vi "hello-vi.vi"() -> ()   [LabVIEW 2020]
uses:
  controls/APC_ControlSettings.ctl
  controls/APC_PIDcontrolSettings.ctl
panel:
  out "System State 2":i8
  in  "stop":bool
  out "Client Connected":bool=TRUE
  out "Telemetry seq":i32
  out "Lines received":i32
  out "Last received":string
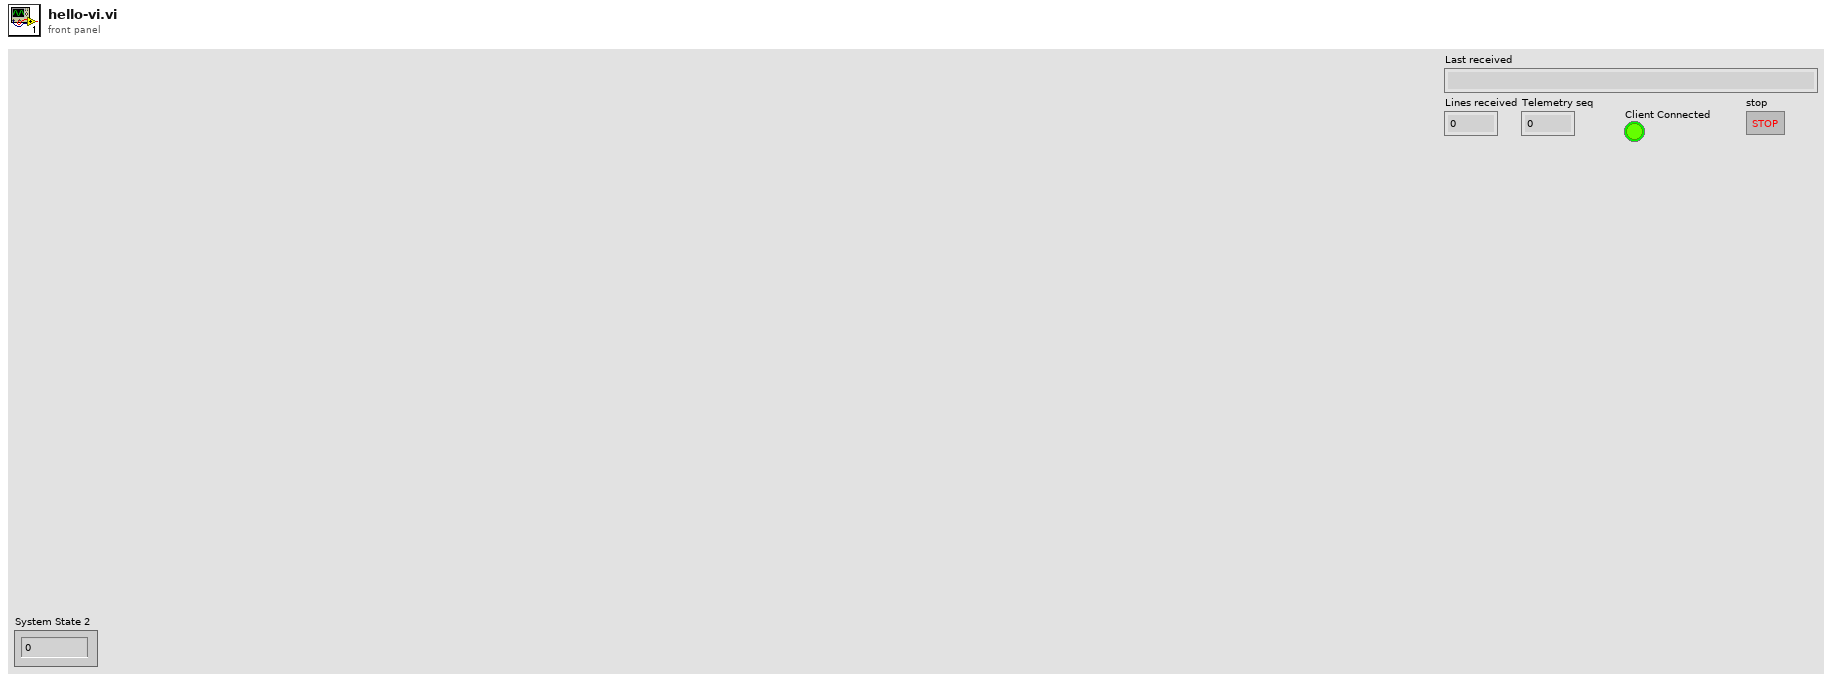
[diagram p1: front panel]
types:
  T1 = enum16{"Standard", "Buffered", "CRLF", "Immediate"}
  T2 = typedef "APC_ControlSettings.ctl" = cluster{"Spark advance [CADBTDC]":dbl, "Pref":dbl, "O2ref":dbl, "DI advance [CADBTDC]":dbl, "DI duration [ms] ":dbl, "CO2ref":dbl, "PFI duration [ms]":dbl, "IMEP ref":dbl, "Speed ref":dbl, "IGN enable":bool, "DI enable":bool, "CL PFI\n lambda":bool, "CL PFI\nIMEP":bool, "Activate\ncylinder":bool[], "Force idling":bool, "Force motoring":bool, "ETP resync":bool, "Requested mode":i8, "Clear Sync Errors":bool, "toggle TDC":bool, "l ref":dbl, "PID control references":T3, "CA50setpoint [CADATDC]":dbl, "CA50 control":bool, "Knock control":bool, "CLEAR EMERGENCY STOP":bool, "EMERGENCY STOP":bool}
  T3 = typedef "APC_PIDcontrolSettings.ctl" = cluster{"NG":bool, "Ar":bool, "O2":bool, "Intake vent":bool, "Cross vent":bool, "Exhaust vent":bool, "NG control mode":u8, "NG-FC-001-REF":dbl, "WF-OA-002-REF":dbl, "IMEP-REF":dbl, "Nm-REF":dbl, "Ar control mode":u8, "AR-PC-002-REF":dbl, "WF-PT-004-REF":dbl, "O2 control mode":u8, "O2-FC-001-REF":dbl, "WF-OA-001-REF":dbl, "Tcoolant control  mode":u8, "EC-FC-001-REF":dbl, "EC-TT-001-REF":dbl, "Texh control mode":u8, "SW-FC-004-REF":dbl, "SW-FT-002-REF":dbl, "WF-TT-004-REF":dbl, "Toil control mode":u8, "SW-FC-009-REF":dbl, "SW-FT-004-REF":dbl, "EO-TT-001-REF":dbl, "AIC201_CO2_ConcTarget":dbl, "O2_FF_NG":bool, "Dyno control mode":u8, "Membrane control mode":u8, "AR-FT-001-REF":dbl, "MTR modbus floats":sgl[], "MTR modbus u16":u16[], "MTR HB":bool, "PC_HB":bool, "EMERGENCY STOP":bool}
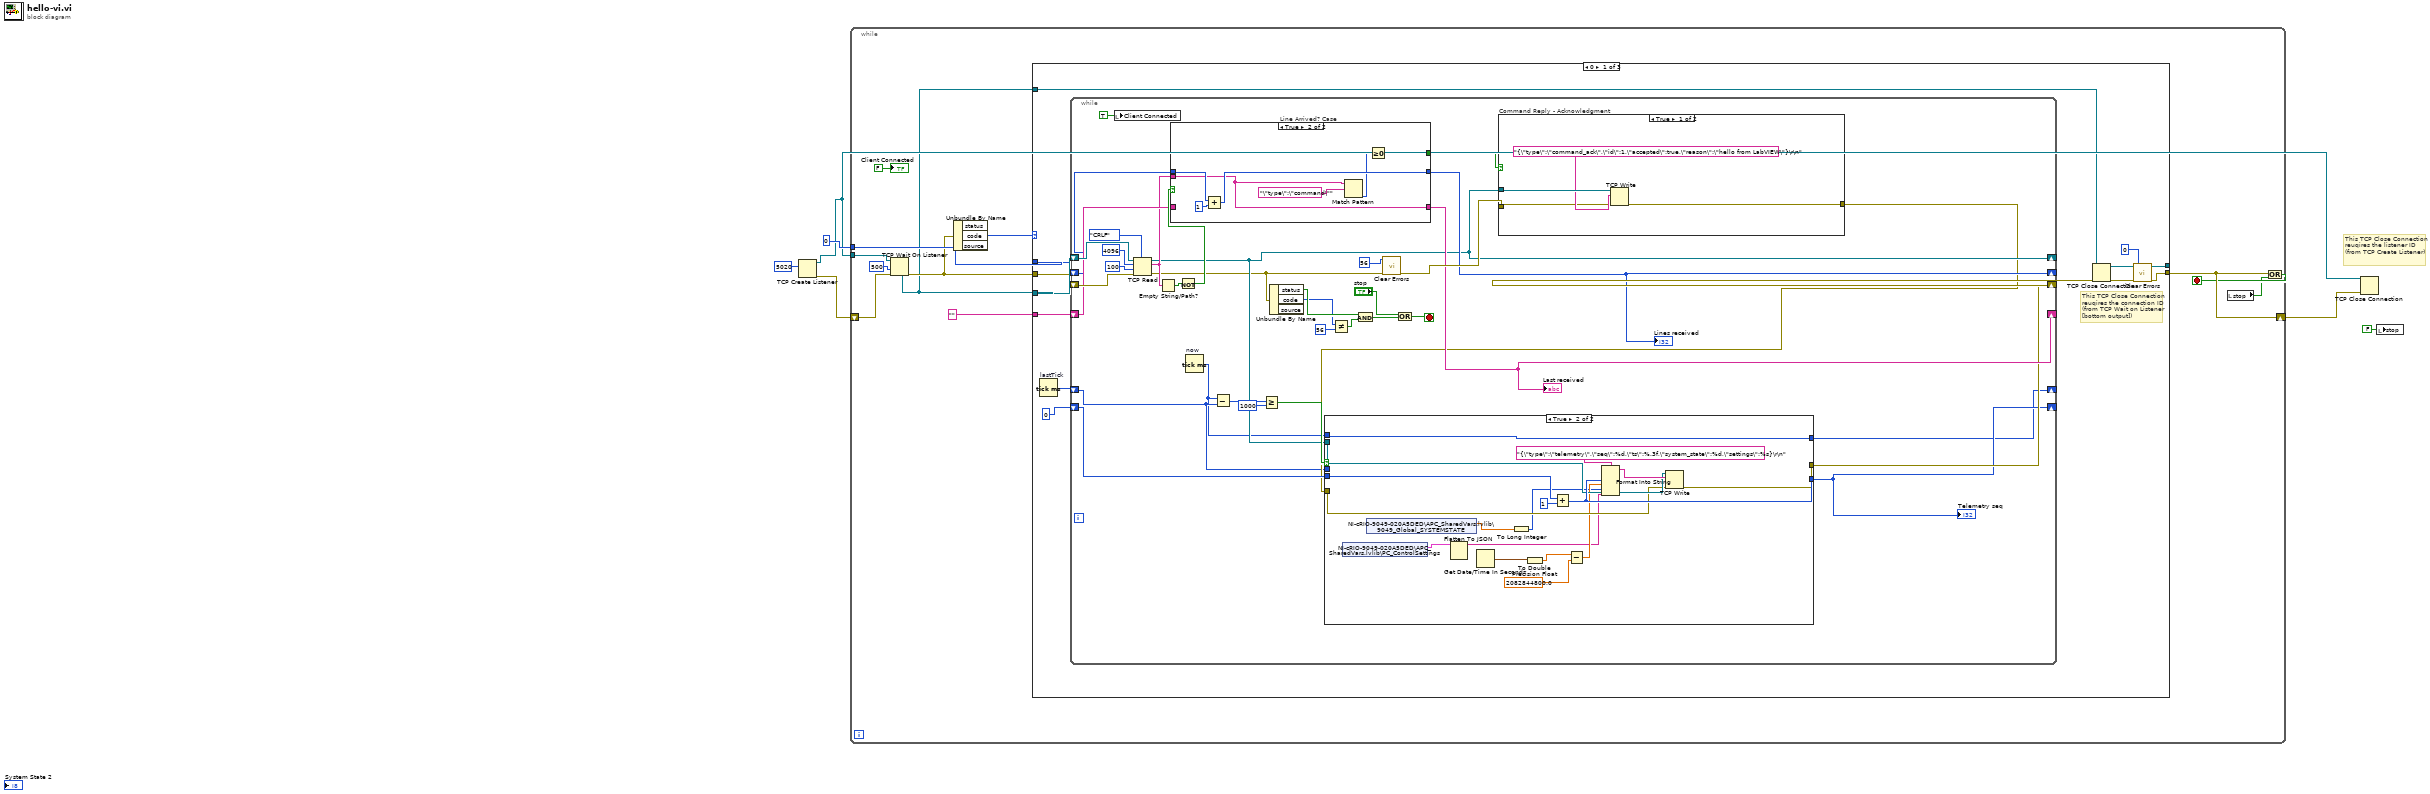
[diagram p0: block diagram]
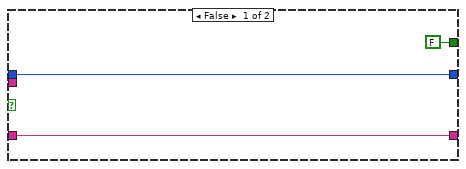
[diagram p3: hidden frame]
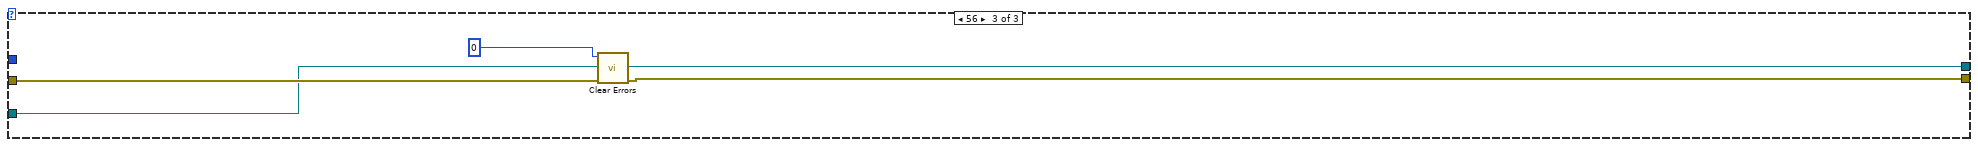
[diagram p6: hidden frame]
diagram:
  # "This TCP Close Connection reuqires the listener ID (from TCP Create Listener)"
  n1 = TCP Create Listener(10:u16 5020 ("port")) -> (0:w4:errorcluster, 3:w1:refnum<k5>)  [unwired: 4 in, 1 out]
  n2 = while {
    tunnel: 0 ("Lines received") -> [w17]
    shift-right: [w12] -> w3
    shift-left: w4 -> [w16]
    tunnel: w1 -> [w9]
    stop <- w11 stop-if-true
    n3 = TCP Wait On Listener(8:w16, 9:500 ("timeout ms (wait forever: -1)"), 11:w9) -> (0:w14:errorcluster, 4:w8:refnum<k5>)  [unwired: 1 in, 3 out]
    n4 = Unbundle By Name(w14) -> ("code"=w13:i32)  [unwired: 2 out]
    n5 = case shown="0" w13 {
      tunnel: w8 -> [w30 w102 w103]
      tunnel: w17 -> [w29 _ _]
      tunnel: [w23 w102 w103] -> _
      tunnel: [w24 w101 w104] -> w12
      tunnel: w14 -> [w28 w101 w105]
      tunnel: w8 -> [w22 _ _]
      tunnel: "" -> [w21 _ _]
      frame 0 {
        # "This TCP Close Connection reuqires the connection ID (from TCP Wait on Listener [bottom output])"
        n6 = Tick Count (ms) "lastTick"() -> (millisecond timer value=w20:u32)
        n7 = while {
          shift-right: [w51] -> _
          shift-left: w29 -> [w52]
          shift-right: [w43] -> w27
          shift-left: w28 -> [w58]
          shift-right: [w45] -> _
          shift-left: w30 -> [w65]
          shift-right: [w53] -> _
          shift-left: w21 -> [w55]
          shift-right: [w41] -> _
          shift-left: w20 -> [w40]
          shift-right: [w42] -> _
          shift-left: 0 -> [w46]
          stop <- w37 stop-if-true
          n8 = local write "Client Connected"(TRUE ("Client Connected")) -> ()
          n9 = TCP Read(connection ID=w65, bytes to read=4096, error in (no error)=w58, 7:T1."CRLF" ("mode (standard)"), 9:100 ("timeout ms (25000)")) -> (connection ID out=w45:refnum<k5>, data out=w54:string, error out=w38:errorcluster)
          n10 = Empty String/Path?(string/path=w54) -> (empty?=w59:bool)
          n11 = Not(x=w59) -> (.not. x?=w56:bool)
          n12 = case "Line Arrived? Case" shown="True" w56 {
            tunnel: w55 -> [w88 _]
            tunnel: [w88 w91] -> w53
            tunnel: w54 -> [_ w91]
            tunnel: w52 -> [w87 w94]
            tunnel: [w87 w93] -> w51
            tunnel: [FALSE w89] -> w50
            frame False {
            }
            frame True {
              n13 = Add(x=w94, y=1) -> (x+y=w93:i32)
              n14 = Match Pattern(string=w91, regular expression="\"type\":\"command\"") -> (offset past match=w90:i32)  [unwired: 1 in, 3 out]
              n15 = Greater Or Equal To 0?(x=w90) -> (x >= 0?=w89:bool)
            }
          }
          "Last received" <- w53
          "Lines received" <- w51
          n16 = Tick Count (ms) "now"() -> (millisecond timer value=w39:u32)
          n17 = Subtract(x=w39, y=w40) -> (x-y=w49:u32)
          n18 = Greater Or Equal?(x=w49, y=u32 1000) -> (x >= y?=w47:bool)
          n19 = Unbundle By Name(w38) -> ("status"=w34:bool, "code"=w33:i32)  [unwired: 1 out]
          n20 = Not Equal?(x=w33, y=56) -> (x != y?=w31:bool)
          n21 = And(x=w34, y=w31) -> (x .and. y?=w35:bool)
          n22 = call <vilib>:"Clear Errors.vi"("error in (no error)"=w38, "specific error code to clear (0: all)"=56) -> ("error out"=w57:errorcluster)  [unwired: 4 in, 1 out]
          n23 = Or(x="stop", y=w35) -> (x .or. y?=w37:bool)
          n24 = case "Command Reply - Acknowledgment" shown="True" w50 {
            tunnel: w45 -> [w99 _]
            tunnel: [w97 w100] -> w44
            tunnel: w57 -> [w96 w100]
            frame True {
              n25 = TCP Write(connection ID=w99, data in="{\"type\":\"command_ack\",\"id\":1,\"accepted\":true,\"reason\":\"hello from LabVIEW\"}\r\n", error in (no error)=w96) -> (error out=w97:errorcluster)  [unwired: 1 in, 2 out]
            }
            frame False {
            }
          }
          n26 = case shown="True" w47 {
            tunnel: w46 -> [w68 w72]
            tunnel: [w68 w83] -> w42
            tunnel: w45 -> [_ w81]
            tunnel: w44 -> [w67 w80]
            tunnel: [w67 w79] -> w43
            tunnel: [w66 w78] -> w41
            tunnel: w40 -> [w66 _]
            tunnel: w39 -> [_ w78]
            frame False {
            }
            frame True {
              n27 = shared-variable "NI-cRIO-9049-020A5DED\\APC_SharedVars.lvlib\\PC_ControlSettings"() -> (w71:T2)  [unwired: 1 in, 1 out]
              n28 = shared-variable "NI-cRIO-9049-020A5DED\\APC_SharedVars.lvlib\\9049_Global_SYSTEMSTATE"() -> (w70:dbl)  [unwired: 1 in, 1 out]
              n29 = Flatten To JSON(anything=w71) -> (JSON string=w73:string)  [unwired: 2 in, 1 out]
              n30 = Get Date/Time In Seconds() -> (seconds since 1Jan1904=w77:timestamp)
              n31 = To Long Integer(number=w70) -> (32bit integer=w69:i32)
              n32 = To Double Precision Float(number=w77) -> (double precision float=w76:dbl)
              n33 = Add(x=w72, y=1) -> (x+y=w83:i32)
              n34 = Subtract(x=w76, y=2082844800.0) -> (x-y=w74:dbl)
              n35 = Format Into String(format string="{\"type\":\"telemetry\",\"seq\":%d,\"ts\":%.3f,\"system_state\":%d,\"settings\":%s}\r\n", w83, w74, w69, w73) -> (resulting string=w82:string)  [unwired: 2 in, 1 out]
              n36 = TCP Write(connection ID=w81, data in=w82, error in (no error)=w80) -> (error out=w79:errorcluster)  [unwired: 1 in, 2 out]
            }
          }
          "Telemetry seq" <- w42
        }
        n37 = TCP Close Connection(connection ID=w22, error in (no error)=w27) -> (connection ID out=w23:refnum<k5>, error out=w26:errorcluster)  [unwired: 1 in]
        n38 = call <vilib>:"Clear Errors.vi"("error in (no error)"=w26, "specific error code to clear (0: all)"=0) -> ("error out"=w24:errorcluster)  [unwired: 4 in, 1 out]
      }
      frame Default {
      }
      frame 56 {
        n39 = call <vilib>:"Clear Errors.vi"("error in (no error)"=w105, "specific error code to clear (0: all)"=0) -> ("error out"=w104:errorcluster)  [unwired: 4 in, 1 out]
      }
    }
    n40 = local read "stop"() -> (w10:bool)
    n41 = Or(x=w12, y=w10) -> (x .or. y?=w11:bool)
    "Client Connected" <- FALSE ("Client Connected")
  }
  n42 = TCP Close Connection(connection ID=w1, error in (no error)=w3) -> ()  [unwired: 1 in, 2 out]
  n43 = local write "stop"(FALSE ("stop")) -> ()
